vi "generate_hear_filter_signal.vi"() -> ()   [LabVIEW 2017]
panel:
  in  "Lower Cut-Off":dbl=100.0
  out "Filtered Signal":dynamicdata(graph)
  out "Frequency":dbl
  out "Amplitude":dbl
  in  "Duration (s)":dbl=1.0
  out "Waveform Graph":dynamicdata(graph)
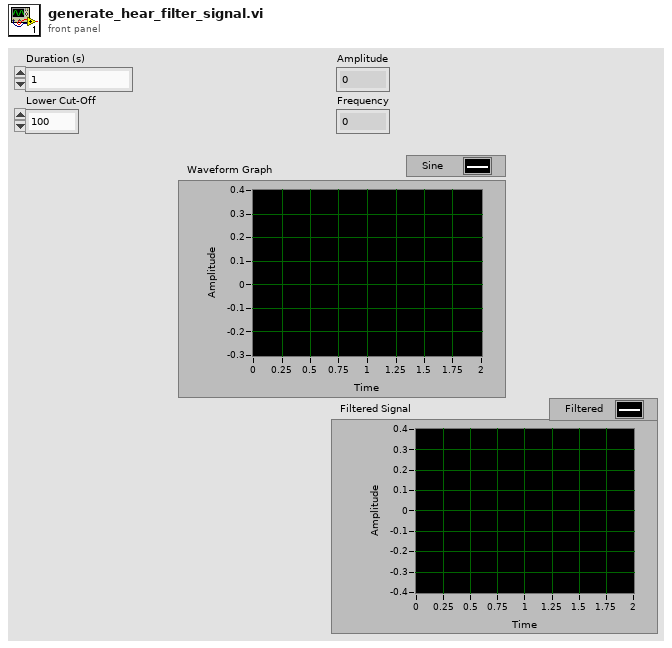
[diagram p1: front panel]
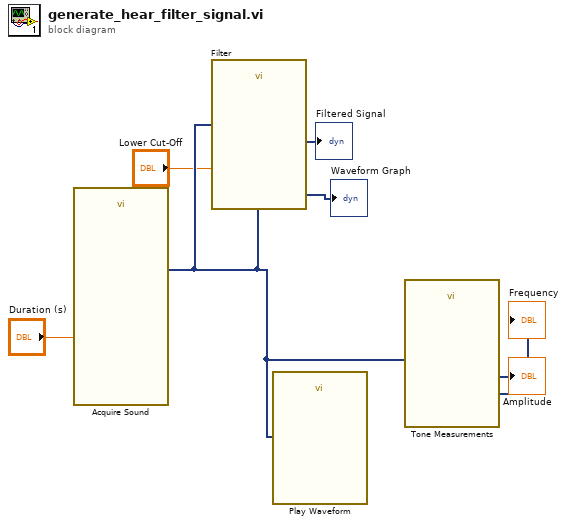
[diagram p0: block diagram]
diagram:
  n1 = call "Acquire Sound"("Duration (s)"="Duration (s)") -> ("Data"=w3:dynamicdata)  [unwired: 17 in, 1 out]
  "Waveform Graph" <- w3
  n2 = call "Filter"("Lower Cut-Off"="Lower Cut-Off", "Signal"=w3) -> ("Filtered Signal"=→"Filtered Signal":dynamicdata)  [unwired: 8 in, 1 out]
  n3 = call "Play Waveform"("Data"=w3) -> ()  [unwired: 18 in, 1 out]
  n4 = call "Tone Measurements"("Signals"=w3) -> ("Frequency"=→"Frequency":dynamicdata, "Amplitude"=→"Amplitude":dynamicdata)  [unwired: 7 in, 2 out]
